vi "sendValue.vi"(8 "error in (no error)":errorcluster, 10 "data":variant, 11 "settingVersions in":refnum<class "settingVersions.lvclass">) -> (0 "error out":errorcluster, 2 "function return":i32, 3 "settingVersions out":refnum<class "settingVersions.lvclass">)   [LabVIEW 2016, in "SALLV_AtDome_Messaging.lvlib" / "settingVersions.lvclass"]
uses:
  settingVersions.lvclass
  ts_sallv_AtDome/DataTypes/logevent_settingVersions.ctl
  settingVersions.lvclass/settingVersions.ctl
  ts_sallv_AtDome/SALLV_AtDome.lvlib
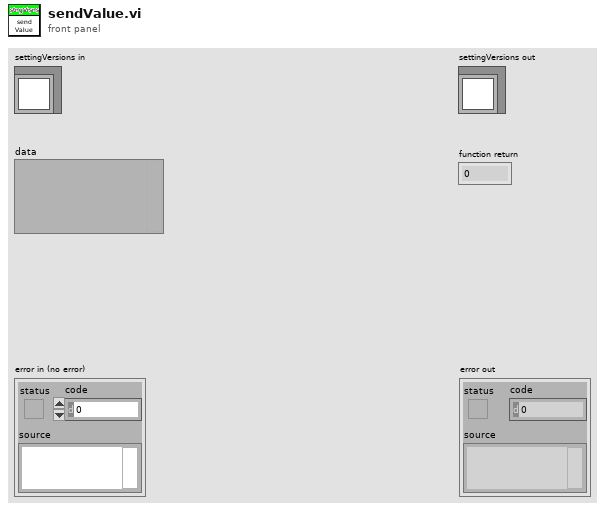
[diagram p1: front panel]
types:
  T1 = typedef "SALLV_AtDome.lvlib/logevent_settingVersions.ctl" = cluster{"recommendedSettingsVersion":string, "recommendedSettingsLabels":string, "priority":i32}
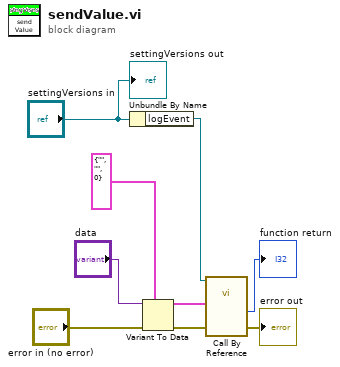
[diagram p0: block diagram]
diagram:
  n1 = Unbundle By Name("settingVersions in") -> ("logEvent"=w7:refnum<vi>)
  n2 = Variant To Data(error in="error in (no error)", type=T1 {"recommendedSettingsVersion"="", "recommendedSettingsLabels"="", "priority"=0} ("logevent_settingVersions"), Variant="data") -> (data=w1:T1, error out=w5:errorcluster)
  n3 = call-by-ref "?"(reference=w7, "error in (no error)"=w5, "logevent_settingVersions_Ctl"=w1) -> ("error out"=→"error out":errorcluster, "function return"=→"function return":i32)  [unwired: 8 in, 3 out]
  "settingVersions out" <- "settingVersions in"
